vi "CameraTest.vi"() -> ()   [LabVIEW 2020]
uses:
  <vilib>/picture/picture.llb/imagedata.ctl
panel:
  out "error out":errorcluster
  out "return value":T1
  out "Numeric":u8
  in  "stop":bool
  out "dt":u32=141
  out "picture":picture
  in  "Camera Params":T2={"plane"="RGB", "zoom"=0.520408163265306, "rotation"=0} {"rotation" scale=0.0..180.0; "zoom" scale=0.0..1.0}
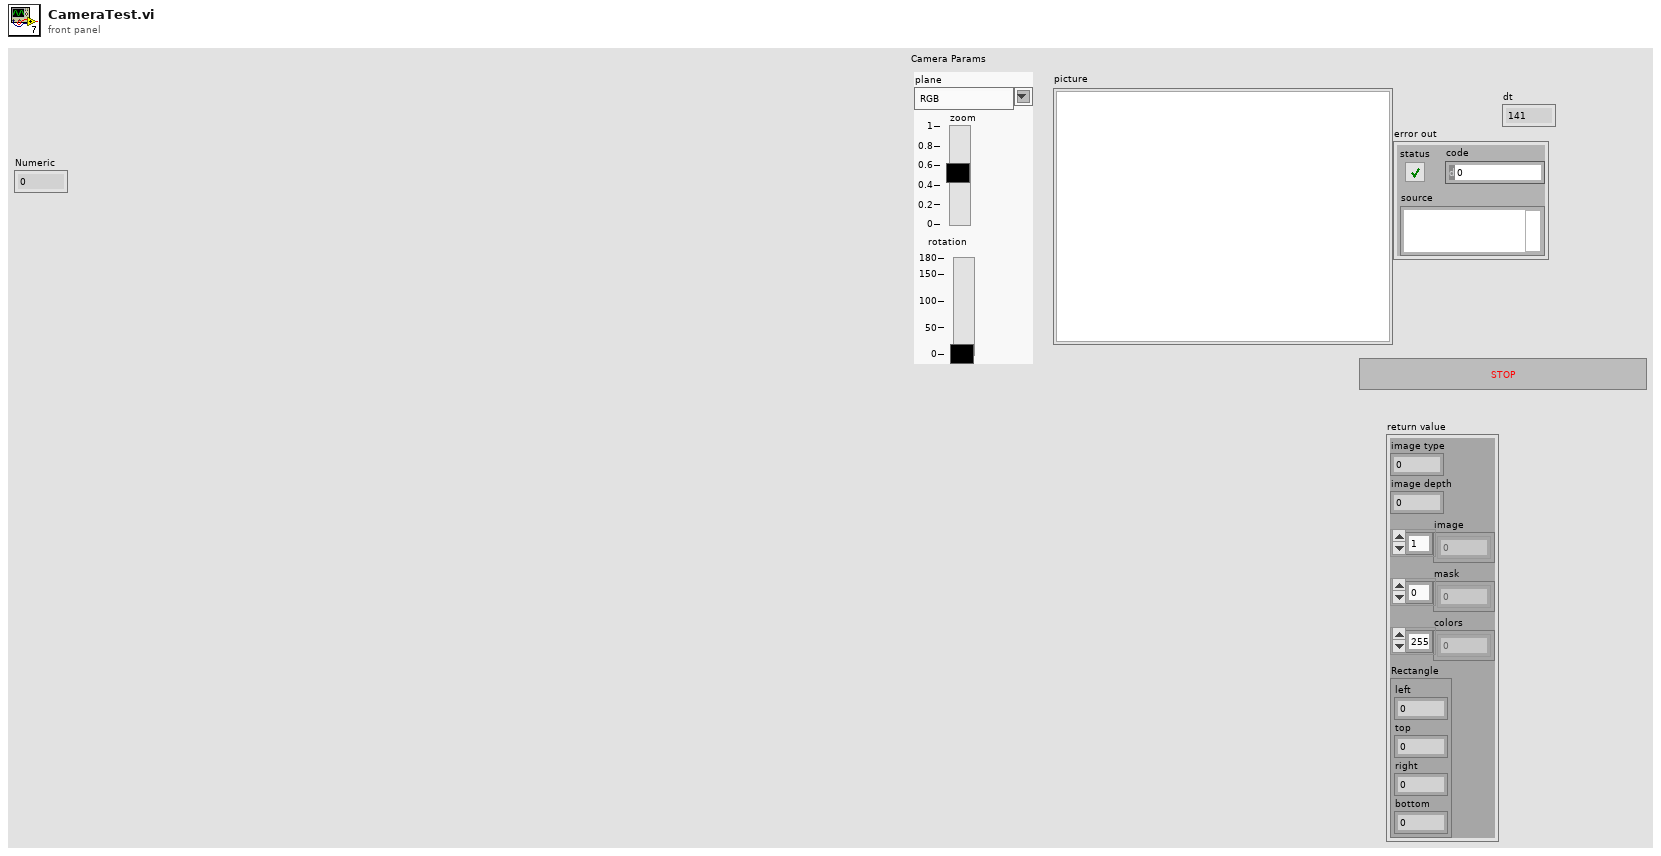
[diagram p1: front panel]
types:
  T1 = typedef "imagedata.ctl" = cluster{"image type":i32, "image depth":i32, "image":u8[], "mask":u8[], "colors":u32[], "Rectangle":cluster{"left":i16, "top":i16, "right":i16, "bottom":i16}}
  T2 = cluster{"plane":string, "zoom":dbl, "rotation":u8}
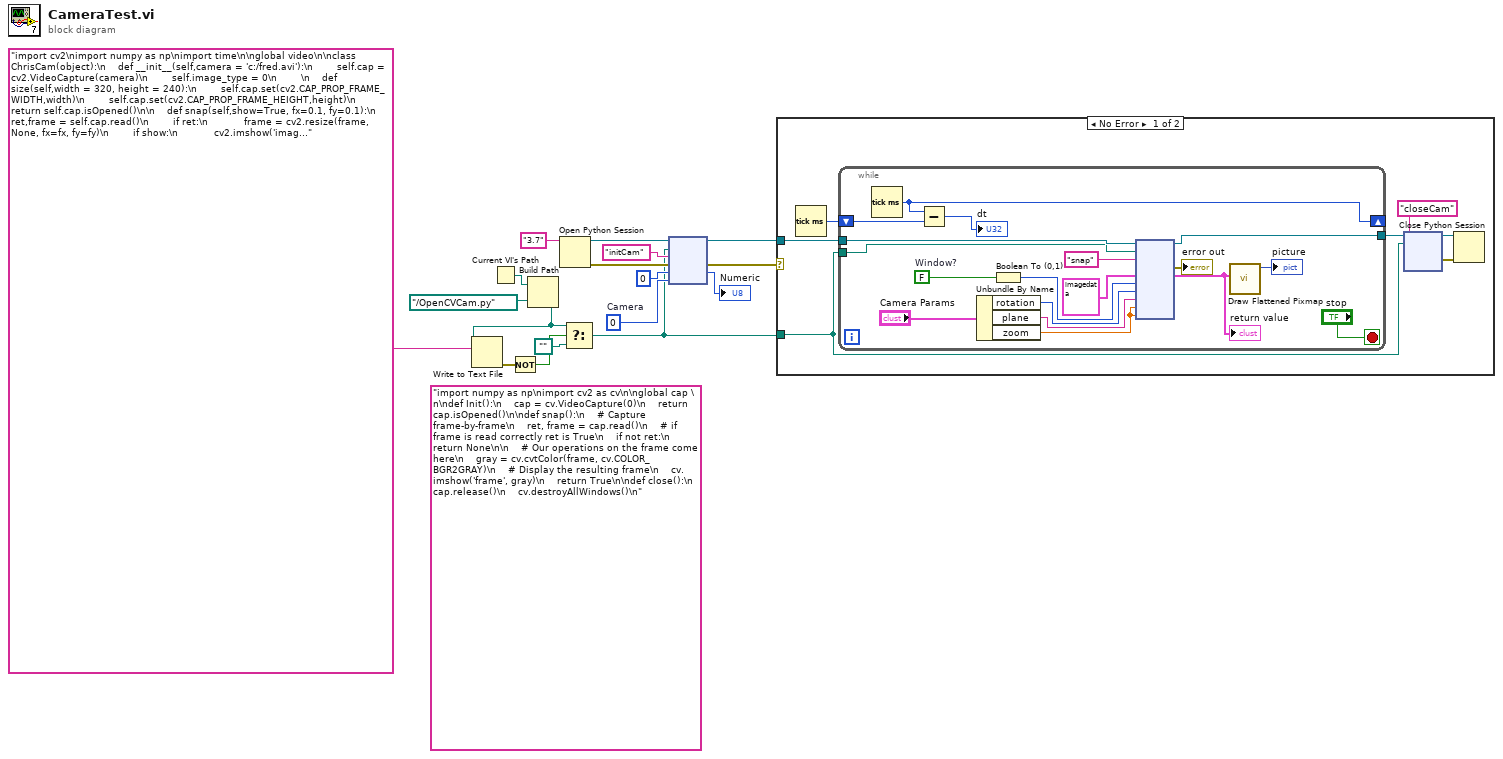
[diagram p0: block diagram]
diagram:
  (unwired) "import numpy as np\nimport cv2 as cv\n\nglobal cap \n\ndef Init():\n    cap = cv.VideoCapture(0)\n    return cap.isOpened()\n\ndef snap():\n    # Capture frame-by-frame\n    ret, frame = cap.read()\n    # if frame is read correctly ret is True\n    if not ret:\n        return None\n\n    # Our operations on the frame come here\n    gray = cv.cvtColor(frame, cv.COLOR_BGR2GRAY)\n    # Display the resulting frame\n    cv.imshow('frame', gray)\n    return True\n\ndef close():\n    cap.release()\n    cv.destroyAllWindows()\n" ("text")
  w16 = 0  # Camera
  n1 = Current VI's Path() -> (path=w6:path)
  n2 = Build Path(base path=w6, name or relative path=path "../OpenCVCam.py") -> (appended path=w15:path)
  n3 = Write to Text File(file (use dialog)=w15, text="import cv2\nimport numpy as np\nimport time\n\nglobal video\n\nclass ChrisCam(object):\n    def __init__(self,camera = 'c:/fred.avi'):\n        self.cap = cv2.VideoCapture(camera)\n        self.image_type = 0\n        \n    def size(self,width = 320, height = 240):\n        self.cap.set(cv2.CAP_PROP_FRAME_WIDTH,width)\n        self.cap.set(cv2.CAP_PROP_FRAME_HEIGHT,height)\n        return self.cap.isOpened()\n\n    def snap(self,show=True, fx=0.1, fy=0.1):\n        ret,frame = self.cap.read()\n        if ret:\n            frame = cv2.resize(frame, None, fx=fx, fy=fy)\n        if show:\n            cv2.imshow('image',frame)\n        return ret, frame\n\n    def rotate(self, img, rotation):\n        rows,cols,depth = img.shape\n        rotationMatrix = cv2.getRotationMatrix2D((cols/2,rows/2),rotation,1)\n        frame = cv2.warpAffine(img,rotationMatrix,(cols,rows))\n        return frame\n\n    def toLV(self,frame,plane = 'RGB'):      # takes around 30 ms per call\n        array = frame.ravel()\n        mask = np.array([])\n        if not plane == 'Gray':\n            image_depth = 24\n            colors = np.array([])\n            fixedFrame = np.empty((array.size,),dtype = array.dtype)\n            if 'R' in plane:\n                fixedFrame[0::3] = array[2::3]   # go from BGR ro RGB\n            if 'G' in plane:\n                fixedFrame[1::3] = array[1::3]\n            if 'B' in plane:\n                fixedFrame[2::3] = array[0::3]\n        else:\n            fixedFrame = np.empty((int(array.size/3),),dtype = array.dtype)\n            fixedFrame[0::1] = array[0::3]# int((int(array[0::3]) + int(array[1::3]) +  int(array[2::3]) ) / 3)\n            image_depth = 8\n            colors = np.array([ (i | i<<8 | i<<16) for i in range(256)])  # define color map\n        self.rectangle = (0,0,frame.shape[1],frame.shape[0])  # this is the LabVIEW rectangle format\n        reply =  (self.image_type, image_depth,fixedFrame.tolist(),mask.tolist(),colors.tolist(),self.rectangle)\n        return reply\n\n    def toCV(self,LVimage):      # takes around 30 ms per call\n        rows,cols = LVimage[5][3],LVimage[5][2]\n        array = np.asarray(LVimage[2],dtype='uint8')\n        fixedFrame = np.empty((array.size,),dtype = array.dtype)\n        fixedFrame[0::3] = array[2::3]   # go from RGB to BGR\n        fixedFrame[1::3] = array[1::3]\n        fixedFrame[2::3] = array[0::3]\n        img = fixedFrame.reshape(rows,cols,3)\n        return img\n\n    def close(self):\n        self.cap.release()\n        cv2.destroyAllWindows()\n        return True\n\ndef initCam(camera = 'c:/fred.avi',width = 640, height = 480):\n    global video\n    video = ChrisCam(camera)\n    return video.size(width,height)\n\ndef snap(show=True, rotation = 90, plane = 'RGB',fx=0.1, fy=0.1):\n    ret, frame = video.snap(show,fx,fy)\n    if not ret:\n        return \n    if not rotation == 0:\n        frame = video.rotate(frame,rotation)\n    return video.toLV(frame,plane)\n\ndef closeCam():\n    return video.close()\n\n") -> (error out=w12:errorcluster)  [unwired: 2 in, 2 out]
  n4 = Not(x=w12) -> (.not. x?=w13:bool)
  n5 = Open Python Session(python version="3.7" ("Python version")) -> (session out=w17:refnum<k35>, error out=w11:errorcluster)  [unwired: 2 in]
  n6 = Select(t=w15, s=w13, f=path "") -> (s? t:f=w1:path)
  n7 = node(w17, w1, "initCam" ("function name"), w11, u8 0, w16) -> (w2:refnum<k35>, w3:errorcluster, →"Numeric":u8)  [unwired: 1 in, 2 out]
  n8 = case shown="No Error" w3 {
    tunnel: w2 -> [w21 _]
    tunnel: w1 -> [w19 _]
    frame No Error {
      n9 = Tick Count (ms)() -> (millisecond timer value=w24:u32)
      n10 = while {
        shift-right: [w42] -> _
        shift-left: w24 -> [w41]
        tunnel: w21 -> [w31]
        tunnel: [w30] -> w20
        tunnel: w19 -> [w29]
        stop <- "stop" stop-if-true
        w32 = FALSE  # Window?
        n11 = Tick Count (ms)() -> (millisecond timer value=w42:u32)
        n12 = Subtract(x=w42, y=w41) -> (x-y=→"dt":u32)
        n13 = Unbundle By Name("Camera Params") -> ("rotation"=w36:u8, "plane"=w35:string, "zoom"=w34:dbl)
        n14 = Boolean To (0,1)(Boolean=w32) -> (0, 1=w37:i16)
        n15 = node(w31, w29, "snap" ("function name"), T1 {"image type"=0, "image depth"=24, "image"=[], "mask"=[], "colors"=[0, 0, 65793, 131586, 197379, 263171, 328965, 394758, 460551, 526344, 592137, 657930, 723723, 789516, 855309, 921102, 986895, 1052688, 1118481, 1184274, 1250067, 1315860, 1381653, 1447446, 1513239, 1579032, 1644825, 1710618, 1776411, 1842204, 1907997, 1973790, 2039583, 2105376, 2171169, 2236962, 2302755, 2368548, 2434341, 2500134, 2565927, 2631720, 2697513, 2763306, 2829099, 2894892, 2960685, 3026478, 3092271, 3158064, 3223857, 3289650, 3355443, 3421236, 3487029, 3552822, 3618615, 3684408, 3750201, 3815994, 3881787, 3947580, 4013373, 4079166, 4144959, 4210752, 4276545, 4342338, 4408131, 4473924, 4539717, 4605510, 4671303, 4737096, 4802889, 4868682, 4934475, 5000268, 5066061, 5131854, 5197647, 5263440, 5329233, 5395026, 5460819, 5526612, 5592405, 5723991, 5789784, 5855577, 5921370, 5987163, 6052956, 6118749, 6184542, 6250335, 6316128, 6381921, 6447714, 6513507, 6579300, 6645093, 6710886, 6776679, 6842472, 6908265, 6974058, 7039851, 7105644, 7171437, 7237230, 7303023, 7368816, 7434609, 7500402, 7566195, 7631988, 7697781, 7763574, 7829367, 7895160, 7960953, 8026746, 8092539, 8158332, 8224125, 8289918, 8355711, 8421504, 8487297, 8553090, 8618883, 8684676, 8750469, 8816262, 8882055, 8947848, 9013641, 9079434, 9145227, 9211020, 9276813, 9342606, 9408399, 9474192, 9539985, 9605778, 9671571, 9737364, 9803157, 9868950, 9934743, 10000536, 10066329, 10132122, 10197915, 10263708, 10329501, 10395294, 10461087, 10526880, 10592673, 10658466, 10724259, 10790052, 10855845, 10921638, 10987431, 11053224, 11119017, 11184810, 11250603, 11382189, 11447982, 11513775, 11579568, 11645361, 11711154, 11776947, 11842740, 11908533, 11974326, 12040119, 12105912, 12171705, 12237498, 12303291, 12369084, 12434877, 12500670, 12566463, 12632256, 12698049, 12763842, 12829635, 12895428, 12961221, 13027014, 13092807, 13158600, 13224393, 13290186, 13355979, 13421772, 13487565, 13553358, 13619151, 13684944, 13750737, 13816530, 13882323, 13948116, 14013909, 14079702, 14145495, 14211288, 14277081, 14342874, 14408667, 14474460, 14540253, 14606046, 14671839, 14737632, 14803425, 14869218, 14935011, 15000804, 15066597, 15132390, 15198183, 15263976, 15329769, 15395562, 15461355, 15527148, 15592941, 15658734, 15724527, 15790320, 15856113, 15921906, 15987699, 16053492, 16119285, 16185078, 16250871, 16316664, 16382457, 16448250, 16514043, 16579836, 16645629, 16711422, 16777215, 16777215], "Rectangle"={"left"=0, "top"=0, "right"=640, "bottom"=480}} ("image data"), w37, w36, w35, w34, w34) -> (w30:refnum<k35>, →"error out":errorcluster, w38:T1)  [unwired: 6 in, 2 out]
        "return value" <- w38
        n16 = call <vilib>:"Draw Flattened Pixmap.vi"("image data"=w38) -> ("new picture"=→"picture":picture)  [unwired: 8 in]
      }
      n17 = node(w20, w19, "closeCam" ("function name")) -> (w22:refnum<k35>, w23:errorcluster)  [unwired: 3 in, 2 out]
      n18 = Close Python Session(session in=w22, error in=w23) -> ()  [unwired: 1 out]
    }
    frame Error {
    }
  }
